vi "MGI Create Directory Chain.vi"(8 "Error In":errorcluster, 10 "File Presence (Auto Detect)":T1, 11 "Path":path) -> (0 "Error Out":errorcluster, 3 "Duplicate Path":path)   [LabVIEW 2020]
doc: "This VI creates any non-existant folders in \"Path\". The \"Auto Detect\" setting of \"File Presence\" searches for a '.' in the name. In this mode a top level folder with a '.' won't get created and a file without an extension will get created as a folder.\n\nAuthored by Robert C. Mortensen\nsupport@mooregoodideas.com\nwww.mooregoodideas.com\n\nCopyright (c) 2010, Moore Good Ideas, Inc.\n\nAll rights reserved.\n\nRedistribution and use in source and binary forms, with or without modification, are permitted provided that the following conditions are met:\n\n * Redistributions of source code must retain the above copyright notice, this list of conditions and the following disclaimer.\n * Redistributions in binary form must reproduce the above copyright notice, this list of conditions and the following disclaimer in the documentation and/or other materials provided with the distribution.\n * Neither the name of Moore Good Ideas, Inc. nor the names of its contributors may be used to endorse or promote products derived from this software without specific prior written permission.\n\nTHIS SOFTWARE IS PROVIDED BY THE COPYRIGHT HOLDERS AND CONTRIBUTORS \"AS IS\" AND ANY EXPRESS OR IMPLIED WARRANTIES, INCLUDING, BUT NOT LIMITED TO, THE IMPLIED WARRANTIES OF MERCHANTABILITY AND FITNESS FOR A PARTICULAR PURPOSE ARE DISCLAIMED. IN NO EVENT SHALL THE COPYRIGHT OWNER OR CONTRIBUTORS BE LIABLE FOR ANY DIRECT, INDIRECT, INCIDENTAL, SPECIAL, EXEMPLARY, OR CONSEQUENTIAL DAMAGES (INCLUDING, BUT NOT LIMITED TO, PROCUREMENT OF SUBSTITUTE GOODS OR SERVICES; LOSS OF USE, DATA, OR PROFITS; OR BUSINESS INTERRUPTION) HOWEVER CAUSED AND ON ANY THEORY OF LIABILITY, WHETHER IN CONTRACT, STRICT LIABILITY, OR TORT (INCLUDING NEGLIGENCE OR OTHERWISE) ARISING IN ANY WAY OUT OF THE USE OF THIS SOFTWARE, EVEN IF ADVISED OF THE POSSIBILITY OF SUCH DAMAGE."
uses:
  MGI Create Directory Chain Behavior Enum.ctl
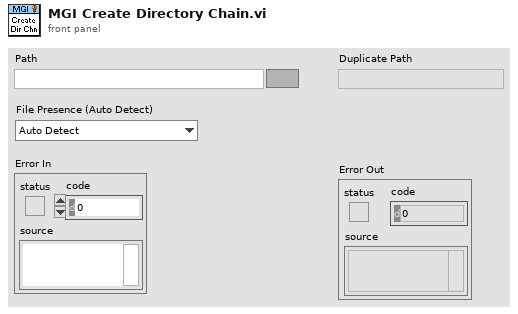
[diagram p1: front panel]
types:
  T1 = typedef "MGI Create Directory Chain Behavior Enum.ctl" = enum16{"Auto Detect", "Path Contains a File", "Path Does Not Contain a File"}
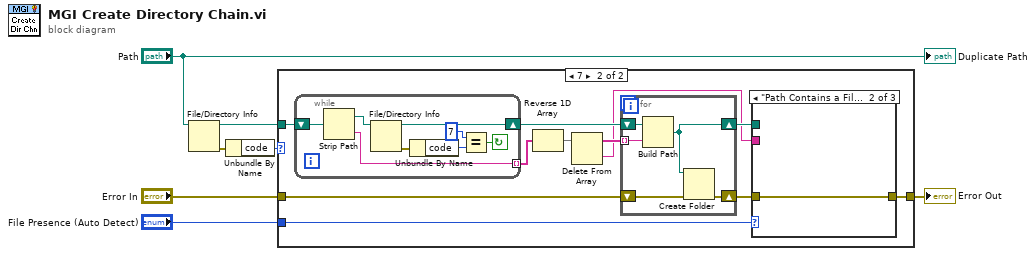
[diagram p0: block diagram]
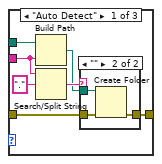
[diagram p3: hidden frame]
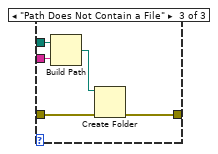
[diagram p5: hidden frame]
diagram:
  n1 = File/Directory Info(path="Path") -> (path out=w2:path, error out=w5:errorcluster)  [unwired: 1 in, 5 out]
  n2 = Unbundle By Name(w5) -> ("code"=w4:i32)
  n3 = case shown="7" w4 {
    tunnel: "Error In" -> [w8 w17]
    tunnel: [w8 w11] -> w7
    tunnel: w2 -> [_ w16]
    tunnel: "File Presence (Auto Detect)" -> [_ w13]
    frame Default {
    }
    frame 7 {
      n4 = while {
        shift-right: [w42] -> w18
        shift-left: w16 -> [w49]
        tunnel: [w43] -> w19 mode=indexing
        stop <- w44 continue-if-true
        n5 = Strip Path(path=w49) -> (stripped path=w48:path, name=w43:string)
        n6 = File/Directory Info(path=w48) -> (path out=w42:path, error out=w47:errorcluster)  [unwired: 1 in, 5 out]
        n7 = Unbundle By Name(w47) -> ("code"=w46:i32)
        n8 = Equal?(x=7 ("y"), y=w46) -> (x = y?=w44:bool)
      }
      n9 = Reverse 1D Array(array=w19) -> (reversed array=w15:string[])
      n10 = Delete From Array(array=w15) -> (deleted portion=w9:string, array with subset deleted=w14:string[])  [unwired: 2 in]
      n11 = for {
        shift-right: [w37] -> w12
        shift-left: w18 -> [w41]
        tunnel: w14 -> [w40] mode=indexing
        shift-right: [w38] -> w10
        shift-left: w17 -> [w39]
        n12 = Build Path(base path=w41, name or relative path=w40) -> (appended path=w37:path)
        n13 = Create Folder(path (use dialog)=w37, error in=w39) -> (error out=w38:errorcluster)  [unwired: 1 in, 2 out]
      }
      n14 = case shown="\"Path Contains a File\"" w13 {
        tunnel: w12 -> [w23 _ w34]
        tunnel: [w20 w31 w35] -> w11
        tunnel: w10 -> [w21 w31 w36]
        tunnel: w9 -> [w22 _ w32]
        frame "Auto Detect" {
          n15 = Build Path(base path=w23, name or relative path=w22) -> (appended path=w25:path)
          n16 = Search/Split String(string=w22, search string/char (-)="." ("search char (-)")) -> (match + rest of string=w26:string)  [unwired: 1 in, 2 out]
          n17 = case shown="\"\"" w26 {
            tunnel: w21 -> [w27 w30]
            tunnel: w25 -> [_ w29]
            tunnel: [w27 w28] -> w20
            frame Default {
            }
            frame "" {
              n18 = Create Folder(path (use dialog)=w29, error in=w30) -> (error out=w28:errorcluster)  [unwired: 1 in, 2 out]
            }
          }
        }
        frame "Path Contains a File" {
        }
        frame "Path Does Not Contain a File" {
          n19 = Build Path(base path=w34, name or relative path=w32) -> (appended path=w33:path)
          n20 = Create Folder(path (use dialog)=w33, error in=w36) -> (error out=w35:errorcluster)  [unwired: 1 in, 2 out]
        }
      }
    }
  }
  "Error Out" <- w7
  "Duplicate Path" <- "Path"
